vi "Flowmeter_Count and Period (Host).vi"() -> ()   [LabVIEW 2013]
doc: "This application runs on the host computer (either RT or Windows) and uses the Count and Period (FPGA) VI for the FPGA Device personality. It demonstrates the RIO board sampling an input for the number of edges over a period of time. The Host VI displays these results and performs additional calculations to determine the frequency of the input signal. This example assumes that the FPGA VI has been compiled for 40MHz in its period calculations."
uses:
  <vilib>/Platform/TimedLoop/XDataNode/timing_clust.ctl
  <vilib>/Platform/TimedLoop/XDataNode/nitl_modes.ctl
  <vilib>/Platform/TimedLoop/XDataNode/wakeup.ctl
  <vilib>/FPGAPlugInAG/myRIO-1900/niLvFpga_Open_myRIO-1900.vi
  <vilib>/Utility/error.llb/Error Cluster From Error Code.vi
  <vilib>/rvi/errors/niLvFpgaAdjustHostInterfaceError.vi
  <vilib>/FPGAPlugInAG/myRIO-1900/niLvFpga_Close_myRIO-1900.vi
  <vilib>/Platform/TimedLoop/XDataNode/XDataNode.xnode
  <vilib>/rvi/interface/nirviOpenFPGA/nirviOpenFPGA.xnode
  FPGA Bitfiles/myRIOAquaponics_FPGATarget_FlowmeterCountan_paXwlCkcw1I.lvbitx
  Flowmeter_Count and Period.vi
  <vilib>/rvi/interface/nirviReadWriteControl/nirviReadWriteControl.xnode
  <vilib>/rvi/interface/nirviCloseFPGA/nirviCloseFPGA.xnode
  <vilib>/Platform/TimedLoop/XDataNode/XDNodeRunTimeDep.lvlib
  NiFpgaLv.dll
panel:
  out "Freq. (Hz)":dbl
  out "FPGA Sampling \nPeriod (ticks)":u32
  out "Host Sampling\nPeriod (sec)":dbl format="%#_3g"
  out "Edge Count":u32
  out "Frequency (Hz)":dbl(knob) caption="Frequency of Digital Signal (Hz)" scale=0.0..500000.0 scale format="%#_4p"
  in  "stop":bool
  # "This VI demonstrates acquiring the number of edges on an input on the FPGA device to determine the frequency of the input signal."
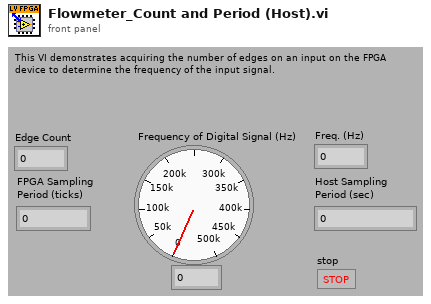
[diagram p1: front panel]
types:
  T1 = typedef "XDNodeRunTimeDep.lvlib/timing_clust.ctl" = cluster{"Expected End [f-1]":u64, "Actual End [f-1]":u64, "Finished Late? [f-1]":bool, "Expected End [i-1]":u64, "Actual End [i-1]":u64, "Finished Late? [i-1]":bool, "Expected Start [i]":u64, "Actual Start [i]":u64, "Expected Start [f]":u64, "Actual Start [f]":u64, "Source Name":string, "Structure Name":string, "Period":i64, "Deadline":i64, "Offset":i64, "Start":i64, "Priority":i32, "Timeout":i32, "Mode":T2, "Wakeup Reason":T3, "Error":errorcluster, "Source Type":string, "Secondary Source Type":string, "Global End Time":u64, "Global Start Time":u64, "Frame Duration":u64, "Iteration Duration":u64, "Assigned CPU":i32, "I/O Scan Engine Mode":u32}
  T2 = typedef "XDNodeRunTimeDep.lvlib/nitl_modes.ctl" = enum32{"No Change", "Process missed periods, maintain original phase", "Discard missed periods, maintain original phase", "Process missed periods, ignore original phase", "Discard missed periods, ignore original phase"}
  T3 = typedef "XDNodeRunTimeDep.lvlib/wakeup.ctl" = enum32{"Normal", "Aborted", "Asynchronous wakeup", "Timing source error", "Timed loop error", "Timeout"}
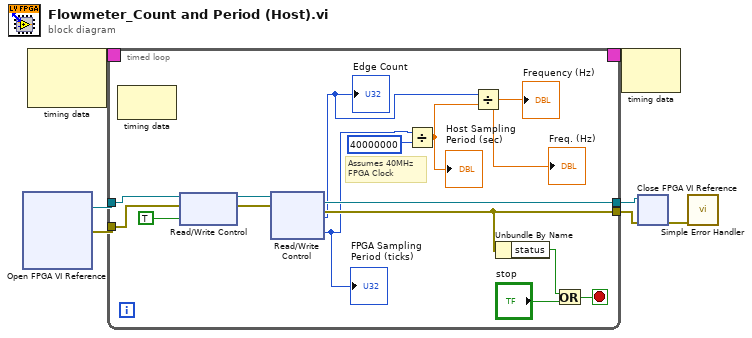
[diagram p0: block diagram]
diagram:
  n1 = xnode "Open FPGA VI Reference"() -> ("FPGA VI Reference Out"=w7:refnum<k20>, "error out"=w6:errorcluster)  [unwired: 2 in]
  n2 = node-c288() -> (w1:T1)  [unwired: 2 out]
  n3 = timed-loop {
    tunnel: [w11] -> w4
    tunnel: [w12] -> w5
    tunnel: w6 -> [w21]
    tunnel: w7 -> [w22]
    timing-out: [_] -> w2
    timing: w1 -> [_]
    stop <- w15 stop-if-true
    # "Assumes 40MHz FPGA Clock"
    n4 = node-c288() -> ()  [unwired: 2 out]
    n5 = xnode "Read/Write Control"("FPGA VI Reference In"=w22, "error in"=w21, "Sample"=TRUE) -> ("FPGA VI Reference Out"=w19:refnum<k20>, "error out"=w18:errorcluster)
    n6 = xnode "Read/Write Control"("FPGA VI Reference In"=w19, "error in"=w18) -> ("FPGA VI Reference Out"=w12:refnum<k20>, "error out"=w11:errorcluster, "Count"=w8:u32, "Period"=w9:u32)
    "Edge Count" <- w8
    "FPGA Sampling \nPeriod (ticks)" <- w9
    n7 = Divide(x=w9, y=40000000) -> (x/y=w13:dbl)
    "Host Sampling\nPeriod (sec)" <- w13
    n8 = Divide(x=w8, y=w13) -> (x/y=→"Frequency (Hz)" →"Freq. (Hz)":dbl)
    n9 = Unbundle By Name(w11) -> ("status"=w17:bool)
    n10 = Or(x=w17, y="stop") -> (x .or. y?=w15:bool)
  }
  n11 = node-c288(w2) -> ()  [unwired: 1 out]
  n12 = xnode "Close FPGA VI Reference"("FPGA VI Reference In"=w5, "error in"=w4) -> ("error out"=w3:errorcluster)
  n13 = call <vilib>:"Simple Error Handler.vi"("error in (no error)"=w3) -> ()  [unwired: 1 in, 8 out]
